vi "Generate Notifier Name.vi"() -> (0 "Notifier Name":string)   [LabVIEW 2015, in "not_Generic Named Notifier.lvlib"]
uses:
  not_Generic Named Notifier.lvlib
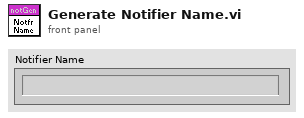
[diagram p1: front panel]
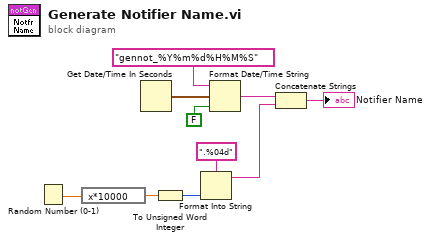
[diagram p0: block diagram]
diagram:
  n1 = Random Number (0-1)() -> (number: 0 to 1=w3:dbl)
  n2 = expression code="x*10000"(w3) -> (w2:dbl)
  n3 = Get Date/Time In Seconds() -> (seconds since 1Jan1904=w9:timestamp)
  n4 = To Unsigned Word Integer(number=w2) -> (unsigned 16bit integer=w1:u16)
  n5 = Format Into String(format string=".%04d", w1) -> (resulting string=w5:string)  [unwired: 2 in, 1 out]
  n6 = Format Date/Time String(time format string (%c)="gennot_%Y%m%d%H%M%S", seconds (now)=w9, UTC format=FALSE) -> (date/time string=w7:string)
  n7 = Concatenate Strings(w7, w5) -> (→"Notifier Name":string)
